vi "read_params.vi"(8 "error in (no error)":errorcluster, 11 "MultiTaskElasticNet in":refnum<class "MultiTaskElasticNet.lvclass">) -> (0 "error out":errorcluster, 2 "params":T1={"alpha"=1.0, "l1_ratio"=0.5, "fit_intercept"=TRUE, "normalize"=FALSE, "copy_X"=TRUE, "max_iter"=1000.0, "tol"=0.0001, "warm_start"=FALSE, "random_state"=0.0, "selection"="cyclic"}, 3 "MultiTaskElasticNet out":refnum<class "MultiTaskElasticNet.lvclass">)   [LabVIEW 2020, in "MultiTaskElasticNet.lvclass"]
uses:
  MultiTaskElasticNet.lvclass
  Controls/multi_task_elastic_net_params.ctl
  MultiTaskElasticNet.lvclass/MultiTaskElasticNet.ctl
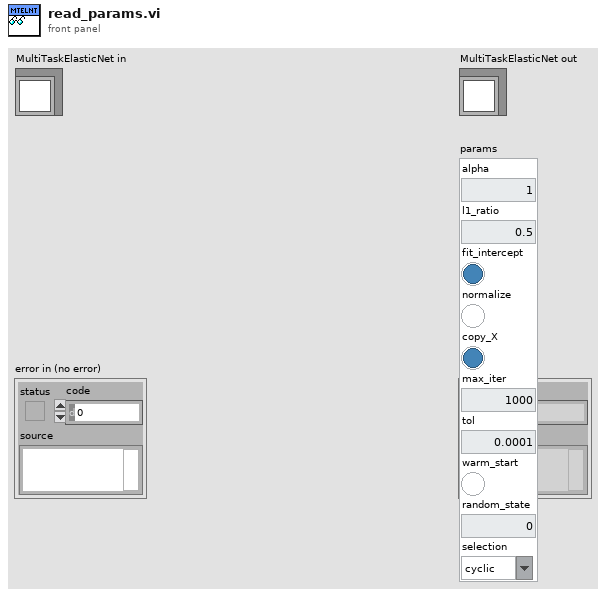
[diagram p1: front panel]
types:
  T1 = typedef "multi_task_elastic_net_params.ctl" = cluster{"alpha":dbl, "l1_ratio":dbl, "fit_intercept":bool, "normalize":bool, "copy_X":bool, "max_iter":dbl, "tol":dbl, "warm_start":bool, "random_state":dbl, "selection":string}
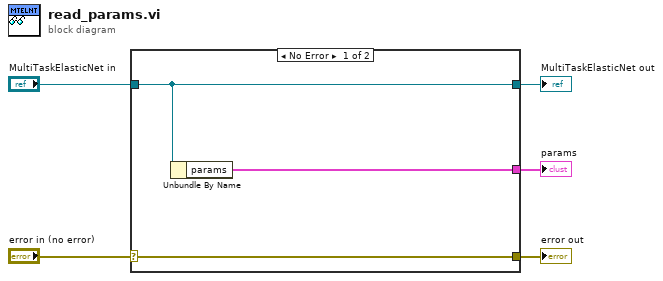
[diagram p0: block diagram]
diagram:
  n1 = case shown="No Error" "error in (no error)" {
    selector: "error in (no error)" -> [w8 w9]
    tunnel: [w8 w9] -> w4
    tunnel: [w7 w10] -> w2
    tunnel: "MultiTaskElasticNet in" -> [w7 w10]
    tunnel: [w6 _] -> w1
    frame No Error {
      n2 = Unbundle By Name(w7) -> ("params"=w6:T1)
    }
    frame Error {
    }
  }
  "error out" <- w4
  "MultiTaskElasticNet out" <- w2
  "params" <- w1
